vi "Get Screw Height (SubVI).vi"(10 "index":i32, 11 "D Array":i16[](array[numeric])) -> (2 "screw_height":dbl[](array[numeric]))   [LabVIEW 2019]
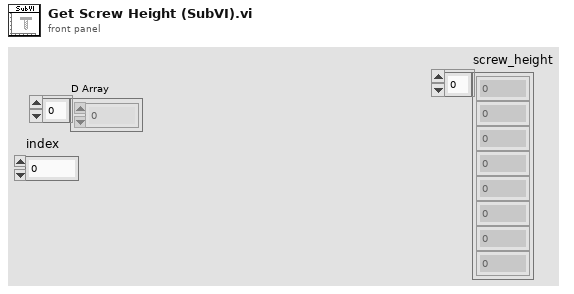
[diagram p1: front panel]
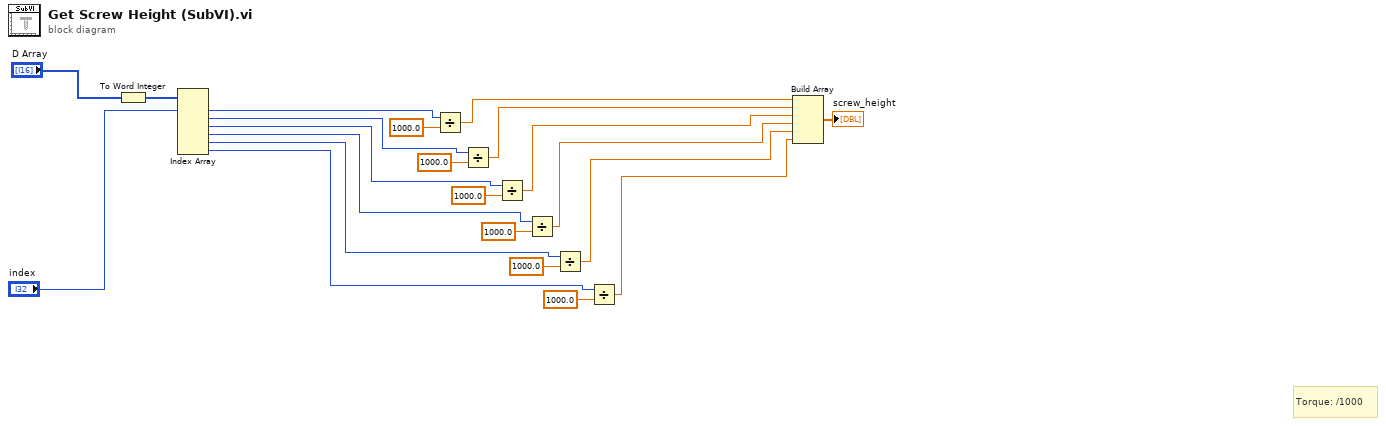
[diagram p0: block diagram]
diagram:
  # "Torque: /1000"
  n1 = To Word Integer(number="D Array") -> (16bit integer=w21:i16[])
  n2 = Index Array(array=w21, index #1="index") -> (element #1=w18:i16, element #2=w16:i16, element #3=w14:i16, element #4=w10:i16, element #5=w9:i16, element #6=w8:i16)  [unwired: 5 in]
  n3 = Divide(x=w18, y=1000.0) -> (x/y=w7:dbl)
  n4 = Divide(x=w16, y=1000.0) -> (x/y=w6:dbl)
  n5 = Divide(x=w14, y=1000.0) -> (x/y=w5:dbl)
  n6 = Divide(x=w10, y=1000.0) -> (x/y=w4:dbl)
  n7 = Divide(x=w9, y=1000.0) -> (x/y=w3:dbl)
  n8 = Divide(x=w8, y=1000.0) -> (x/y=w2:dbl)
  n9 = Build Array(w7, w6, w5, w4, w3, w2) -> (→"screw_height":dbl[])
